vi "fxpRemoveLater.vi"() -> ()   [LabVIEW 2018]
uses:
  <vilib>/rvi/Emulation/niFpgaGetClockAttributes.vi
  <vilib>/rvi/Emulation/niFpgaSctlEmulationGetInTimedLoop.vi
  <vilib>/rvi/Emulation/niFpgaEmulationReportErrorSimple.vi
  <vilib>/rvi/Emulation/niFpgaCriticalErrorInLSC.vi
panel:
  out "binary I16":i16 format="%b"
  out "binary U16":u16 format="%b"
  in  "stop":bool
  out "integer I16":i16
  out "integer U16":u16
  out "Boolean array":bool[](array[boolean])
  out "unsigned 16bit integer":u16
  in  "integer 16":i16
  in  "Mod2 NI-9221":fxp<+/-,16,7> format="%#_8g"
  in  "Mod1 NI-9201":fxp<+/-,16,5> format="%b"
  out "integer to fxp 3":fxp<+/-,16,7> format="%#_8g"
  out "fxp to integer 3":i16
  out "integer to fxp 2":fxp<+/-,16,5> format="%#_8g"
  out "fxp to integer 2":i16
  # "https://knowledge.ni.com/KnowledgeArticleDetails?id=kA03q000000x4XbCAI&l=en-US"
  # "https://www.ni.com/docs/en-US/bundle/labview/page/lvconcepts/numeric_data.html#:~:text=Word%20length%E2%80%94The%20total%20number,word%20length%20of%2064%20bits."
  # "https://www.ni.com/docs/en-US/bundle/labview-fpga-module/page/lvfpgaconcepts/fpgafixedpoint.html"
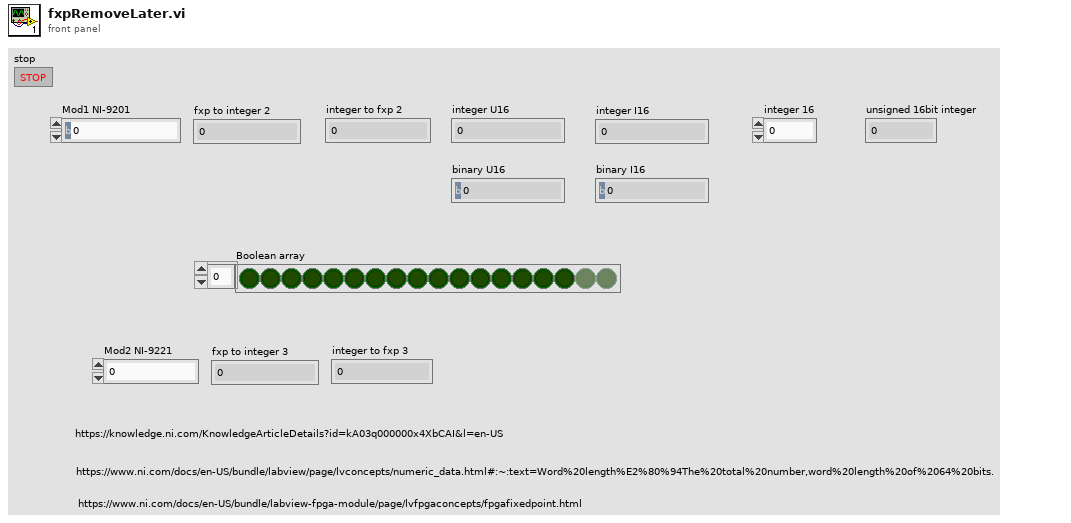
[diagram p1: front panel]
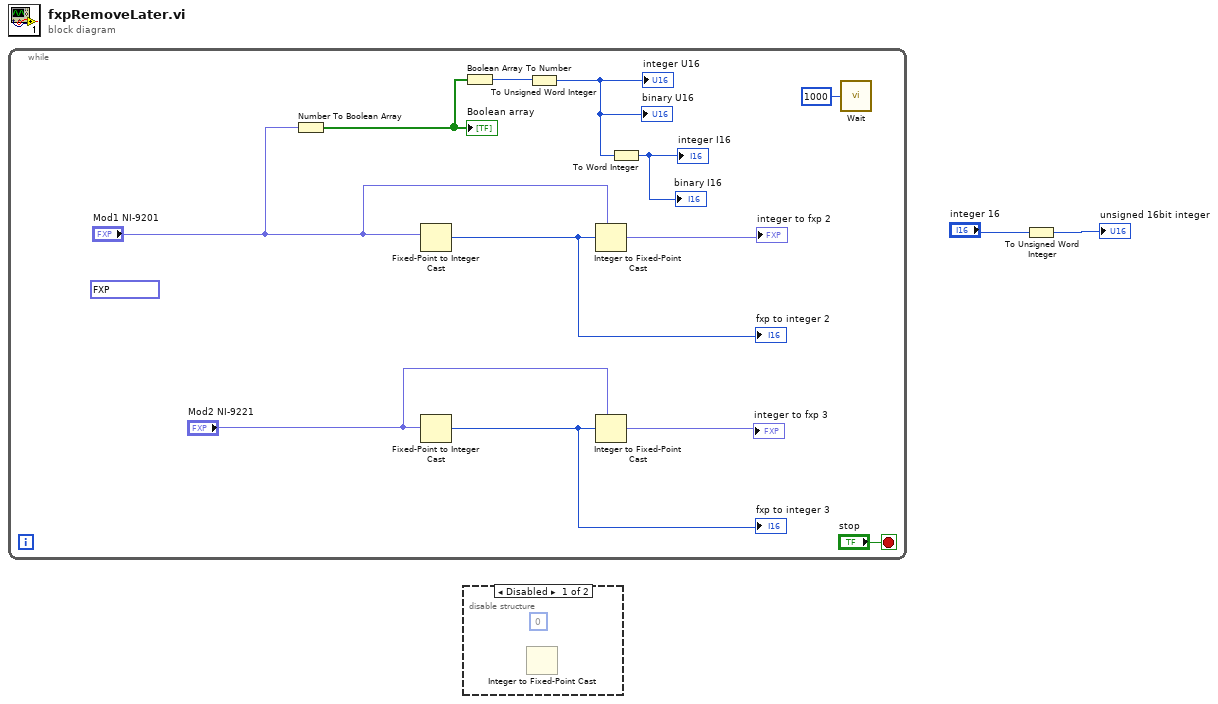
[diagram p0: block diagram]
diagram:
  n1 = while {
    stop <- "stop" stop-if-true
    (unwired) fxp<+/-,16,5> 0.00048828125 ("Mod1 NI-9201")
    n2 = Number To Boolean Array(number="Mod1 NI-9201") -> (Boolean array=w9:bool[])
    "Boolean array" <- w9
    n3 = Fixed-Point to Integer Cast(1:"Mod1 NI-9201") -> (0:w14:i16)
    "fxp to integer 2" <- w14
    n4 = Fixed-Point to Integer Cast(1:"Mod2 NI-9221") -> (0:w11:i16)
    "fxp to integer 3" <- w11
    n5 = Boolean Array To Number(Boolean array=w9) -> (number=w8:u16)
    n6 = To Unsigned Word Integer(number=w8) -> (unsigned 16bit integer=w7:u16)
    "integer U16" <- w7
    "binary U16" <- w7
    n7 = Integer to Fixed-Point Cast(fixed-point type="Mod1 NI-9201", integer=w14) -> (fixed-point=→"integer to fxp 2":fxp<+/-,16,5>)
    n8 = Integer to Fixed-Point Cast(fixed-point type="Mod2 NI-9221", integer=w11) -> (fixed-point=→"integer to fxp 3":fxp<+/-,16,7>)
    n9 = To Word Integer(number=w7) -> (16bit integer=→"integer I16" →"binary I16":i16)
    n10 = call "Wait"("Count(mSec)"=u32 1000) -> ()  [unwired: 1 out]
  }
  n11 = disable-structure shown="Disabled" {
    frame Disabled {
      (unwired) i16 0
      n12 = Integer to Fixed-Point Cast() -> ()  [unwired: 2 in, 1 out]
    }
    frame Enabled {
    }
  }
  n13 = To Unsigned Word Integer(number="integer 16") -> (unsigned 16bit integer=→"unsigned 16bit integer":u16)
